vi "Downable.vi"(1 "输入":dbl[][](array[numeric]), 2 "Bottom":dbl, 3 "y":dbl) -> (0 "输出":bool)   [LabVIEW 2016]
panel:
  out "数值":dbl
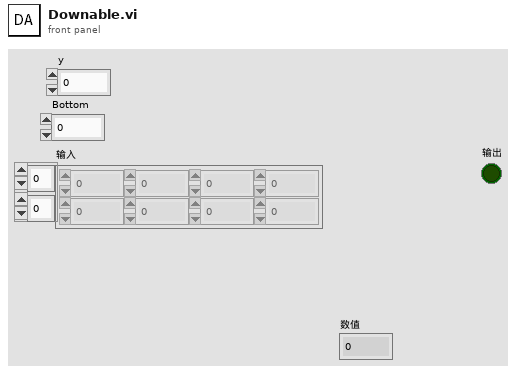
[diagram p1: front panel]
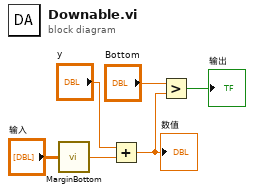
[diagram p0: block diagram]
diagram:
  n1 = call "MarginBottom.vi"("输入"="输入") -> ("输出"=w4:dbl)
  n2 = Add(x="y", y=w4) -> (x+y=w2:dbl)
  "数值" <- w2
  n3 = Greater?(x="Bottom", y=w2) -> (0:→"输出":bool)
